vi "TensionerPositionControl.vi"(11 "Buttons":bool[](array[boolean])) -> ()   [LabVIEW 2015]
uses:
  Utilities/MotorPositionGlobals.vi
panel:
  in  "TensionerSetpoint":dbl=-400000.0 format="%#_13g"
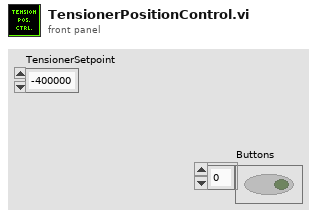
[diagram p1: front panel]
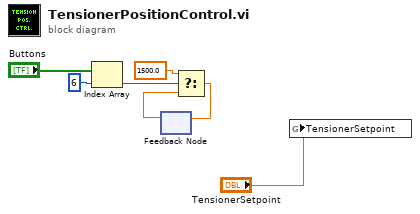
[diagram p0: block diagram]
diagram:
  n1 = Index Array(array="Buttons", index=6) -> (element=w5:bool)
  n2 = feedback #1() -> (w3:dbl)  [unwired: 1 in]
  n3 = Select(t=1500.0, s=w5, f=w3) -> (s? t:f=w2:dbl)
  n4 = feedback-in #1(w2) -> ()
  n5 = global write "MotorPositionGlobals.vi" "TensionerSetpoint"("TensionerSetpoint") -> ()
